vi "PalmSense Read Config File.vi"(7 "configuration file path":path=path "PSConf.ini") -> (0 "error out":errorcluster)   [LabVIEW 2020]
uses:
  support/PCT FGV CMD.ctl
  <vilib>/Utility/config.llb/Read Key (Double).vi
  <vilib>/Utility/config.llb/NI_LVConfig.lvlib
  <vilib>/Utility/config.llb/Write Key (String).vi
  <vilib>/regexp/Match Regular Expression.xnode
  <vilib>/Utility/config.llb/Write Key (Path).vi
  <vilib>/Utility/config.llb/Write Key (Double).vi
  <vilib>/Utility/config.llb/Write Key (Boolean).vi
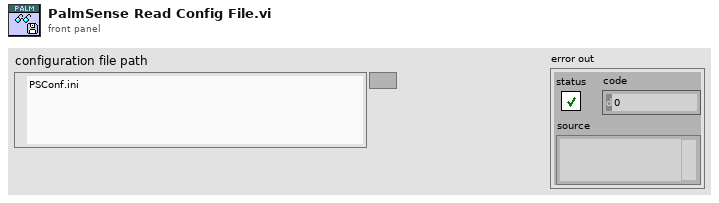
[diagram p1: front panel]
types:
  T1 = typedef "PCT FGV CMD.ctl" = enum16{"INIT", "GET", "SET"}
  T2 = typedef "NI_LVConfig.lvlib/Config Data RefNum.ctl" = refnum<k1>
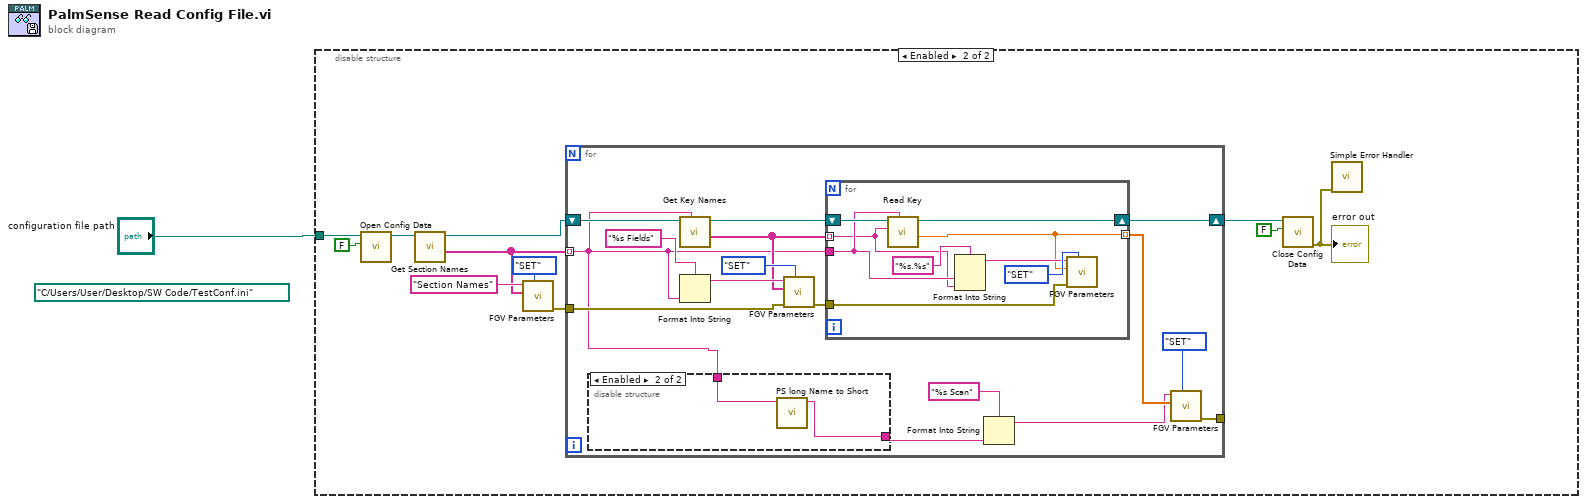
[diagram p0: block diagram]
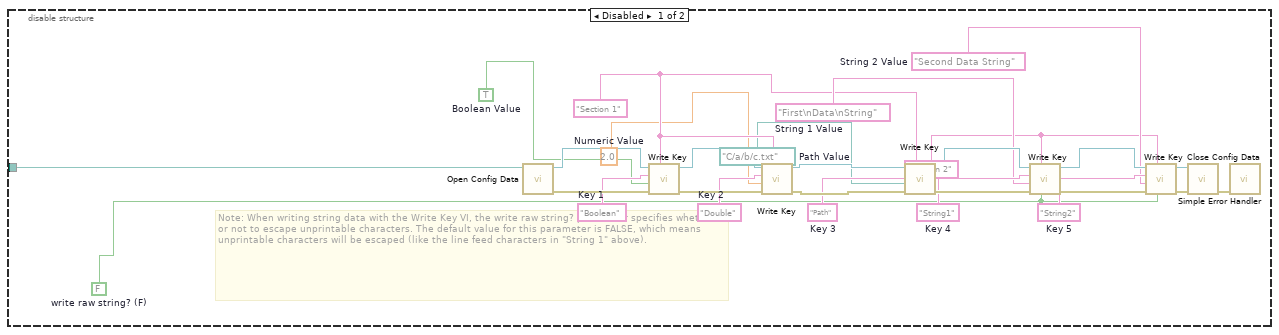
[diagram p2: hidden frame]
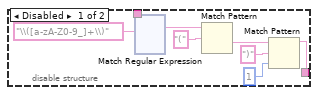
[diagram p3: hidden frame]
diagram:
  (unwired) path "C:/Users/User/Desktop/SW Code/TestConf.ini" ("configuration file path")
  n1 = disable-structure shown="Enabled" {
    disable-tunnel: "configuration file path" -> [w2 w36]
    frame Disabled {
      w10 = "Second Data String"  # String 2 Value
      w11 = "First\nData\nString"  # String 1 Value
      w6 = path "C:/a/b/c.txt"  # Path Value
      w5 = 2.0  # Numeric Value
      w4 = TRUE  # Boolean Value
      w3 = FALSE  # write raw string? (F)
      w12 = "String2"  # Key 5
      w13 = "String1"  # Key 4
      w14 = "Path"  # Key 3
      w15 = "Double"  # Key 2
      w16 = "Boolean"  # Key 1
      w7 = "Section 2"
      w8 = "Section 1"
      # "Note: When writing string data with the Write Key VI, the write raw string? parameter specifies whether or not to escape unprintable characters. The default value for this parameter is FALSE, which means unprintable characters will be escaped (like the line feed characters in \"String 1\" above)."
      n2 = call <vilib>:"Open Config Data.vi"("configuration file path"=w2) -> ("error out"=w22:errorcluster, "refnum"=w28:T2)  [unwired: 2 in, 7 out]
      n3 = call-poly <vilib>:"Write Key.vi"("section"=w8, "error in (no error)"=w22, "value"=w4, "key"=w16, "refnum"=w28) -> ("error out"=w21:errorcluster, "refnum out"=w27:T2)  [unwired: 5 out]
      n4 = call-poly <vilib>:"Write Key.vi"("section"=w8, "error in (no error)"=w21, "value"=w5, "key"=w15, "refnum"=w27) -> ("error out"=w20:errorcluster, "refnum out"=w26:T2)  [unwired: 3 in, 2 out]
      n5 = call-poly <vilib>:"Write Key.vi"("section"=w8, "error in (no error)"=w20, "value"=w6, "key"=w14, "refnum"=w26) -> ("error out"=w19:errorcluster, "refnum out"=w25:T2)  [unwired: 5 out]
      n6 = call-poly <vilib>:"Write Key.vi"("write raw string? (F)"=w3, "section"=w7, "error in (no error)"=w19, "value"=w11, "key"=w13, "refnum"=w25) -> ("error out"=w18:errorcluster, "refnum out"=w24:T2)  [unwired: 4 out]
      n7 = call-poly <vilib>:"Write Key.vi"("write raw string? (F)"=w3, "section"=w7, "error in (no error)"=w18, "value"=w10, "key"=w12, "refnum"=w24) -> ("error out"=w17:errorcluster, "refnum out"=w23:T2)  [unwired: 4 out]
      n8 = call <vilib>:"Close Config Data.vi"("error in (no error)"=w17, "refnum"=w23) -> ("error out"=w9:errorcluster)  [unwired: 1 in, 8 out]
      n9 = call <vilib>:"Simple Error Handler.vi"("error in (no error)"=w9) -> ()  [unwired: 1 in, 8 out]
    }
    frame Enabled {
      n10 = call <vilib>:"Open Config Data.vi"("create file if necessary (T)"=FALSE ("create file if necessary? (T)"), "configuration file path"=w36) -> ("refnum"=w35:T2)  [unwired: 7 in, 2 out]
      n11 = call <vilib>:"Get Section Names.vi"("refnum"=w35) -> ("section names"=w31:string[], "refnum out"=w34:T2)  [unwired: 8 in, 1 out]
      n12 = call "FGV Parameters.vi"("CMD"=PCT_FGV_CMD."SET", "input"=w31, "Key"="Section Names") -> ("error out"=w29:errorcluster)  [unwired: 6 in, 2 out]
      n13 = for {
        tunnel: w31 -> [w45] mode=indexing
        shift-right: [w53] -> w33
        shift-left: w34 -> [w55]
        tunnel: w29 -> [w51]
        tunnel: [w40] -> _
        n14 = disable-structure shown="Enabled" {
          disable-tunnel: w45 -> [w57 w179]
          disable-tunnel: [w56 w178] -> w44
          frame Disabled {
            n15 = xnode "Match Regular Expression"("input string"=w57, "regular expression"="\\([a-zA-Z0-9_]+\\)") -> ("whole match"=w60:string)  [unwired: 4 in, 4 out]
            n16 = Match Pattern(string=w60, regular expression="(") -> (after substring=w58:string)  [unwired: 1 in, 3 out]
            n17 = Match Pattern(string=w58, regular expression=")", offset (0)=1) -> (before substring=w56:string)  [unwired: 3 out]
          }
          frame Enabled {
            n18 = call "PS long Name to Short.vi"("String"=w179) -> ("whole match"=w178:string)  [unwired: 10 in]
          }
        }
        n19 = call <vilib>:"Get Key Names.vi"("section"=w45, "refnum"=w55) -> ("key names"=w48:string[], "refnum out"=w54:T2)  [unwired: 6 in, 2 out]
        n20 = Format Into String(format string="%s Fields", w45) -> (resulting string=w49:string)  [unwired: 2 in, 1 out]
        n21 = call "FGV Parameters.vi"("CMD"=PCT_FGV_CMD."SET", "error in (no error)"=w51, "input"=w48, "Key"=w49) -> ("error out"=w47:errorcluster)  [unwired: 5 in, 2 out]
        n22 = for {
          tunnel: w45 -> [w185]
          tunnel: w48 -> [w184] mode=indexing
          shift-right: [w187] -> w53
          shift-left: w54 -> [w188]
          tunnel: w47 -> [w181]
          tunnel: [w180] -> w43 mode=indexing
          n23 = call-poly <vilib>:"Read Key.vi"("section"=w185, "key"=w184, "refnum"=w188) -> ("value"=w180:dbl, "refnum out"=w187:T2)  [unwired: 2 in, 5 out]
          n24 = Format Into String(format string="%s.%s", w185, w184) -> (resulting string=w182:string)  [unwired: 2 in, 1 out]
          n25 = call "FGV Parameters.vi"("CMD"=PCT_FGV_CMD."SET", "error in (no error)"=w181, "input"=w180, "Key"=w182) -> ()  [unwired: 5 in, 3 out]
        }
        n26 = Format Into String(format string="%s Scan" ("Key"), w44) -> (resulting string=w41:string)  [unwired: 2 in, 1 out]
        n27 = call "FGV Parameters.vi"("CMD"=PCT_FGV_CMD."SET", "input"=w43, "Key"=w41) -> ("error out"=w40:errorcluster)  [unwired: 6 in, 2 out]
      }
      n28 = call <vilib>:"Close Config Data.vi"("write file if changed (T)"=FALSE ("write configuration file? (T)"), "refnum"=w33) -> ("error out"=w37:errorcluster)  [unwired: 1 in, 8 out]
      "error out" <- w37
      n29 = call <vilib>:"Simple Error Handler.vi"("error in (no error)"=w37) -> ()  [unwired: 1 in, 8 out]
    }
  }
